vi "Close.vi"(8 "error in (no error)":errorcluster, 11 "Concrete.lvlib:Hioki9002.lvclass":refnum<class "Hioki9002.lvclass">) -> (0 "error out":errorcluster, 3 "Concrete.lvlib:Hioki9002.lvclass 2":refnum<class "Hioki9002.lvclass">)   [LabVIEW 2021, in "Concrete.lvlib" / "Hioki9002.lvclass"]
uses:
  Hioki9002.lvclass
  Hioki9002.lvclass/Hioki9002.ctl
  Harware Abstraction/Switch/Switch.lvclass
  <instrlib>/HIOKI SW100X Series/HIOKI SW100X Series.lvlib
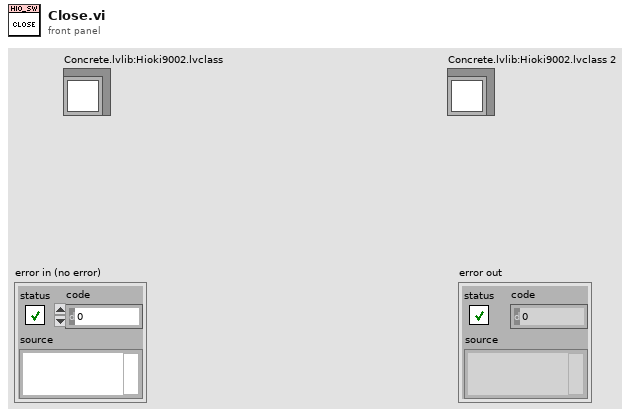
[diagram p1: front panel]
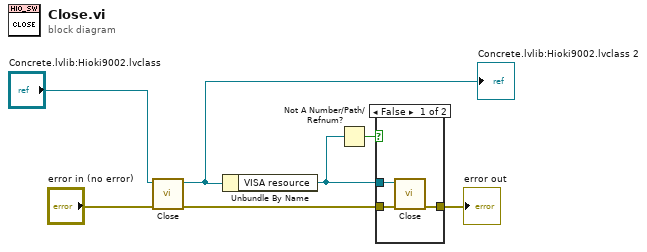
[diagram p0: block diagram]
diagram:
  n1 = call-parent <instrlib>:"Close.vi"("error in (no error)"="error in (no error)", "Instrument in"="Concrete.lvlib:Hioki9002.lvclass") -> ("error out"=w6:errorcluster, "Instrument out"=w1:refnum<class "Hioki9002.lvclass">)  [unwired: 8 in]
  "Concrete.lvlib:Hioki9002.lvclass 2" <- w1
  n2 = Unbundle By Name(w1) -> ("VISA resource"=w4:refnum<visa-resource-name>)
  n3 = Not A Number/Path/Refnum?(number/path/refnum=w4) -> (NaN/Path/Refnum?=w3:bool)
  n4 = case shown="False" w3 {
    tunnel: w6 -> [w10 w11]
    tunnel: [w9 w11] -> w5
    tunnel: w4 -> [w8 _]
    frame False {
      n5 = call <instrlib>:"Close.vi"("error in (no error)"=w10, "VISA resource name"=w8) -> ("error out"=w9:errorcluster)  [unwired: 9 in]
    }
    frame True {
    }
  }
  "error out" <- w5
